vi "VI_ProcessUSerCommands.vi"(8 "error in (no error)":errorcluster, 10 "send command":string, 11 "Common Refs":T1={"LBox_ChList"=refnum, "OXY_SCPI Ref"="TCPIP0::192.168.1.75::10001::SOCKET", "STR_ChName1"=refnum, "STR_ChName2"=refnum, "STR_ChName3"=refnum, "STR_ChName4"=refnum, "STR_ChName5"=refnum, "STR_ChName6"=refnum, "Button_Stop"=refnum, "Button_Start"=refnum, "Button_Disconnect"=refnum, "Button_Connect"=refnum, "Bool_StatusLED"=refnum, "DS Ref"="TCPIP0::192.168.1.75::10001::SOCKET", "Button_SetPort"=refnum, "Button_GetPort"=refnum, "Button_GetState"=refnum, "Button_Reset"=refnum, "Button_Init"=refnum, "STR_UserCMD"=refnum, "STR_CmdPromp"=refnum, "Port"=refnum, "Button_QuerryChs"=refnum, "Graph"=refnum, "STR_ConnAddress"=refnum}) -> (0 "error out":errorcluster, 3 "Common Refs 2":T1={"LBox_ChList"=refnum, "OXY_SCPI Ref"="TCPIP0::192.168.1.75::10001::SOCKET", "STR_ChName1"=refnum, "STR_ChName2"=refnum, "STR_ChName3"=refnum, "STR_ChName4"=refnum, "STR_ChName5"=refnum, "STR_ChName6"=refnum, "Button_Stop"=refnum, "Button_Start"=refnum, "Button_Disconnect"=refnum, "Button_Connect"=refnum, "Bool_StatusLED"=refnum, "DS Ref"="TCPIP0::192.168.1.75::10001::SOCKET", "Button_SetPort"=refnum, "Button_GetPort"=refnum, "Button_GetState"=refnum, "Button_Reset"=refnum, "Button_Init"=refnum, "STR_UserCMD"=refnum, "STR_CmdPromp"=refnum, "Port"=refnum, "Button_QuerryChs"=refnum, "Graph"=refnum, "STR_ConnAddress"=refnum})   [LabVIEW 2020]
uses:
  TypeDefs/Refs_Common.ctl
  TypeDefs/Enum_CmdPromptActions.ctl
  <vilib>/Stadlmann TEC/OXYGEN Datastream/OXYGEN_Datastream.lvlib
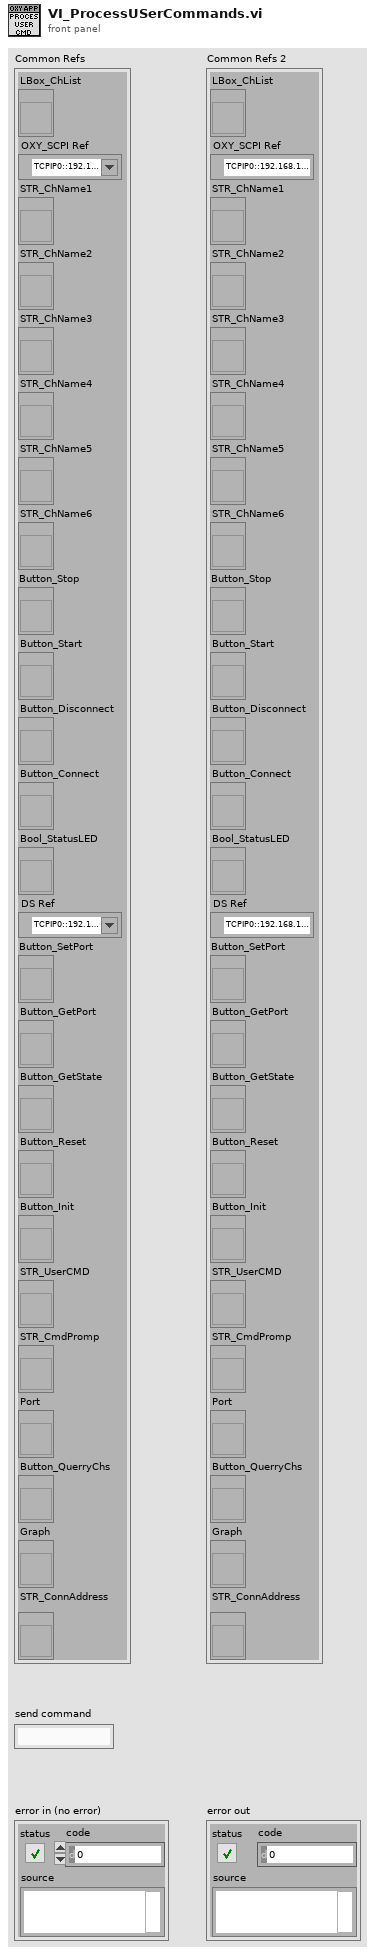
[diagram p1: front panel]
types:
  T1 = typedef "Refs_Common.ctl" = cluster{"LBox_ChList":refnum<vi>, "OXY_SCPI Ref":refnum<visa-resource-name>, "STR_ChName1":refnum<vi>, "STR_ChName2":refnum<vi>, "STR_ChName3":refnum<vi>, "STR_ChName4":refnum<vi>, "STR_ChName5":refnum<vi>, "STR_ChName6":refnum<vi>, "Button_Stop":refnum<vi>, "Button_Start":refnum<vi>, "Button_Disconnect":refnum<vi>, "Button_Connect":refnum<vi>, "Bool_StatusLED":refnum<vi>, "DS Ref":refnum<visa-resource-name>, "Button_SetPort":refnum<vi>, "Button_GetPort":refnum<vi>, "Button_GetState":refnum<vi>, "Button_Reset":refnum<vi>, "Button_Init":refnum<vi>, "STR_UserCMD":refnum<vi>, "STR_CmdPromp":refnum<vi>, "Port":refnum<vi>, "Button_QuerryChs":refnum<vi>, "Graph":refnum<vi>, "STR_ConnAddress":refnum<vi>}
  T2 = typedef "Enum_CmdPromptActions.ctl" = enum16{"Init", "Add", "EditSettings", "Close"}
  T3 = typedef "OXYGEN_Datastream.lvlib/Cluster_RawCommData.ctl" = cluster{"send_data":string, "received_data":string}
  T4 = typedef "OXYGEN_Datastream.lvlib/States.ctl" = enum16{"Invalid", "Config", "Initialized", "Running", "Error", "Unlicensed"}
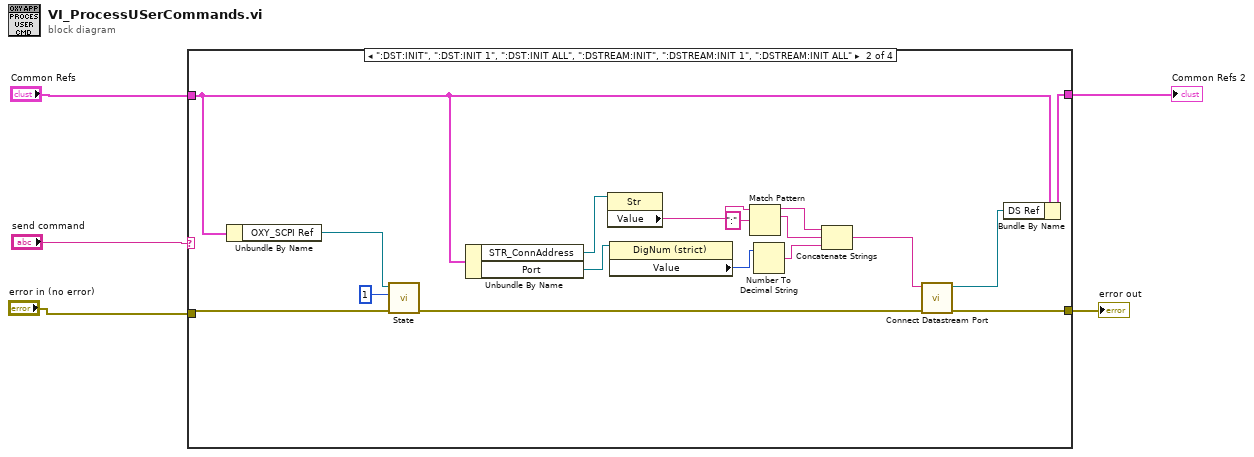
[diagram p0: block diagram]
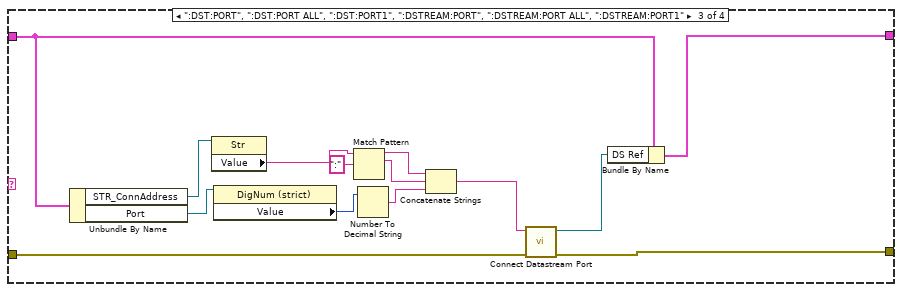
[diagram p3: hidden frame]
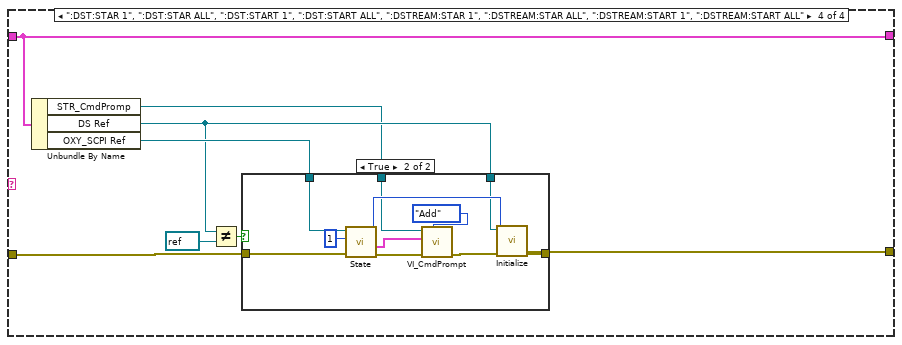
[diagram p4: hidden frame]
diagram:
  n1 = case shown="\":DST:INIT\", \":DST:INIT 1\", \":DST:INIT ALL\", \":DSTREAM:INIT\", \":DSTREAM:INIT 1\", \":DSTREAM:INIT ALL\"" "send command" {
    tunnel: "Common Refs" -> [w6 w8 w30 w44]
    tunnel: "error in (no error)" -> [w7 w23 w27 w46]
    tunnel: [w7 w9 w28 w45] -> w2
    tunnel: [w6 w10 w29 w44] -> w1
    frame Default {
    }
    frame ":DST:INIT", ":DST:INIT 1", ":DST:INIT ALL", ":DSTREAM:INIT", ":DSTREAM:INIT 1", ":DSTREAM:INIT ALL" {
      n2 = Unbundle By Name(w8) -> ("OXY_SCPI Ref"=w22:refnum<visa-resource-name>)
      n3 = call <vilib>:"State.vi"("error in (no error)"=w23, "Group"=1, "OXY_SCPI Reseource In"=w22) -> ("error out"=w11:errorcluster)  [unwired: 5 in, 3 out]
      n4 = Unbundle By Name(w8) -> ("STR_ConnAddress"=w15:refnum<vi>, "Port"=w20:refnum<vi>)
      n5 = property class="Str"(reference=w15) -> ("Value"=w14:string)  [unwired: 1 in, 2 out]
      n6 = property class="DigNum (strict)"(reference=w20) -> ("Value"=w19:u32)  [unwired: 1 in, 2 out]
      n7 = Match Pattern(string=w14, regular expression=":") -> (before substring=w18:string, match substring=w17:string)  [unwired: 1 in, 2 out]
      n8 = Number To Decimal String(number=w19) -> (decimal integer string=w16:string)  [unwired: 1 in]
      n9 = Concatenate Strings(w18, w17, w16) -> (w13:string)
      n10 = call <vilib>:"Connect Datastream Port.vi"("error in (no error)"=w11, "OXY_SCPI Resource In"=w13) -> ("error out"=w9:errorcluster, "OXY_SCPI Resource Out"=w12:refnum<visa-resource-name>)  [unwired: 8 in]
      n11 = Bundle By Name(cluster=w8, "DS Ref"=w12) -> (w10:T1)
    }
    frame ":DST:PORT", ":DST:PORT ALL", ":DST:PORT1", ":DSTREAM:PORT", ":DSTREAM:PORT ALL", ":DSTREAM:PORT1" {
      n12 = Unbundle By Name(w30) -> ("STR_ConnAddress"=w32:refnum<vi>, "Port"=w37:refnum<vi>)
      n13 = property class="Str"(reference=w32) -> ("Value"=w31:string)  [unwired: 1 in, 2 out]
      n14 = property class="DigNum (strict)"(reference=w37) -> ("Value"=w36:u32)  [unwired: 1 in, 2 out]
      n15 = Match Pattern(string=w31, regular expression=":") -> (before substring=w35:string, match substring=w34:string)  [unwired: 1 in, 2 out]
      n16 = Number To Decimal String(number=w36) -> (decimal integer string=w33:string)  [unwired: 1 in]
      n17 = Concatenate Strings(w35, w34, w33) -> (w26:string)
      n18 = call <vilib>:"Connect Datastream Port.vi"("error in (no error)"=w27, "OXY_SCPI Resource In"=w26) -> ("error out"=w28:errorcluster, "OXY_SCPI Resource Out"=w25:refnum<visa-resource-name>)  [unwired: 8 in]
      n19 = Bundle By Name(cluster=w30, "DS Ref"=w25) -> (w29:T1)
    }
    frame ":DST:STAR 1", ":DST:STAR ALL", ":DST:START 1", ":DST:START ALL", ":DSTREAM:STAR 1", ":DSTREAM:STAR ALL", ":DSTREAM:START 1", ":DSTREAM:START ALL" {
      n20 = Unbundle By Name(w44) -> ("STR_CmdPromp"=w39:refnum<vi>, "DS Ref"=w40:refnum<visa-resource-name>, "OXY_SCPI Ref"=w41:refnum<visa-resource-name>)
      n21 = Not Equal?(x=w40, y=refnum<visa-resource-name> refnum) -> (x != y?=w42:bool)
      n22 = case shown="True" w42 {
        tunnel: w46 -> [w47 w54]
        tunnel: [w47 w58] -> w45
        tunnel: w41 -> [_ w56]
        tunnel: w40 -> [_ w55]
        tunnel: w39 -> [_ w48]
        frame False {
        }
        frame True {
          n23 = call <vilib>:"State.vi"("error in (no error)"=w54, "Group"=1, "OXY_SCPI Reseource In"=w56) -> ("error out"=w51:errorcluster, "communication_data"=w50:T3, "State"=w57:T4)  [unwired: 5 in, 1 out]
          n24 = call "VI_CmdPrompt.vi"("Mode"=Enum_CmdPromptActions."Add", "error in (no error)"=w51, "communication_data"=w50, "STR_CmdPrompt_Ref"=w48) -> ("error out"=w49:errorcluster)  [unwired: 7 in]
          n25 = call <vilib>:"Initialize.vi"("error in (no error)"=w49, "Datastrem State"=w57, "OXY_SCPI Resource In"=w55) -> ("error out"=w58:errorcluster)  [unwired: 7 in, 1 out]
        }
      }
    }
  }
  "error out" <- w2
  "Common Refs 2" <- w1
